vi "1chFFT.vi"(4 "Array":dbl[](array[numeric]) caption="X", 5 "频率":dbl) -> (0 "频谱图":dbl[](graph), 2 "幅度值":dbl)   [LabVIEW 2014]
uses:
  <vilib>/Analysis/2dsp.llb/Real FFT.vi
  <vilib>/Analysis/NI_AALPro.lvlib
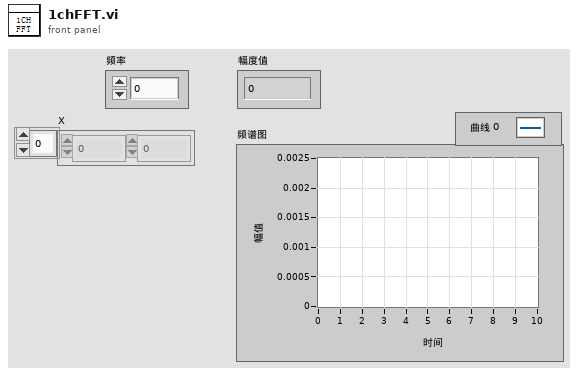
[diagram p1: front panel]
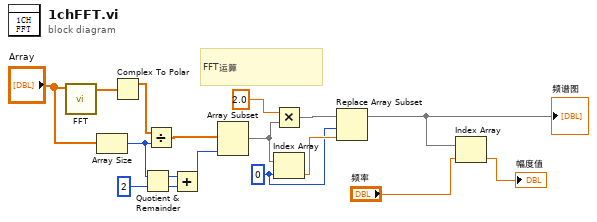
[diagram p0: block diagram]
diagram:
  w8 = 0 ("索引")
  # "FFT运算"
  n1 = call-poly <vilib>:"FFT.vi"("X"="Array") -> ("FFT {X}"=w17:cdb[])  [unwired: 9 in, 1 out]
  n2 = Array Size(array="Array") -> (size(s)=w6:i32)
  n3 = Complex To Polar(r * e^(i*theta)=w17) -> (r=w16:dbl[])  [unwired: 1 out]
  n4 = Quotient & Remainder(x=w6, y=2) -> (x-y*floor(x/y)=w14:i32, floor(x/y)=w15:i32)
  n5 = Divide(x=w16, y=w6) -> (x/y=w7:dbl[])
  n6 = Add(x=w14, y=w15) -> (x+y=w13:i32)
  n7 = Array Subset(array=w7, length=w13) -> (w11:dbl[])  [unwired: 1 in]
  n8 = Multiply(x=2.0, y=w11) -> (x*y=w9:dbl[])
  n9 = Index Array(array=w11, index=w8) -> (element=w10:dbl)
  n10 = Replace Array Subset(array=w9, new element=w10, index=w8) -> (w4:dbl[])
  "频谱图" <- w4
  n11 = Index Array(array=w4, index="频率") -> (element=→"幅度值":dbl)
